vi "Create Queue Dev#3(DP05104B).vi"(8 "error in":errorcluster) -> (0 "error out":errorcluster, 3 "queDev#3":refnum<queue>)   [LabVIEW 2016]
uses:
  Library/Event/Ctl/EventVariantData.ctl
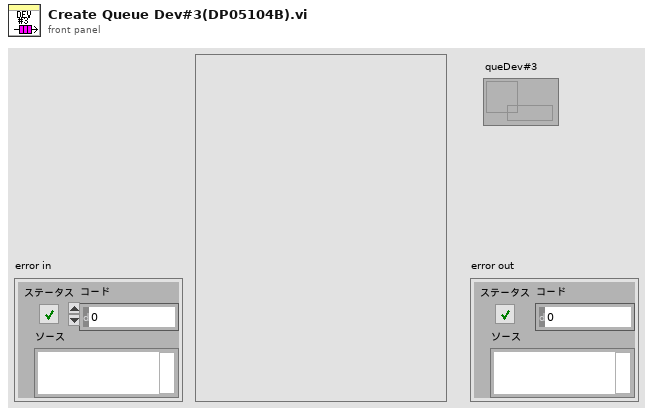
[diagram p1: front panel]
types:
  T1 = typedef "EventVariantData.ctl" = cluster{"コマンド":string, "バリアント":variant}
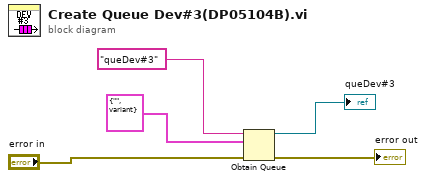
[diagram p0: block diagram]
diagram:
  n1 = Obtain Queue(name (unnamed)="queDev#3" ("名前（名前なし）"), element data type=T1 {"コマンド"="", "バリアント"=variant}, error in (no error)="error in") -> (queue out=→"queDev#3":refnum<queue>, error out=→"error out":errorcluster)  [unwired: 2 in, 1 out]
